vi "Sub Routing program.vi"(4 "Load Graph":refnum<vi>, 5 "Image":refnum<vi>, 6 "Test Name":refnum<vi>, 7 "FeedBack Channel":string[](array[string]), 8 "error in (no error)":errorcluster, 9 "Feature Step Enable":T1(array[cluster]), 10 "Table":refnum<vi>, 11 "queue Out in":refnum<queue>) -> (0 "error out":errorcluster, 1 "Error":bool, 2 "reference out":refnum<vi>, 3 "Queue out":refnum<queue>)   [LabVIEW 2015]
uses:
  Test  enqueue/AutoTest seq.ctl
  Galobal variable_TI.vi
panel:
  out "2D Picture 2":picture
  out "error out 2":errorcluster
  out "2D Picture":picture
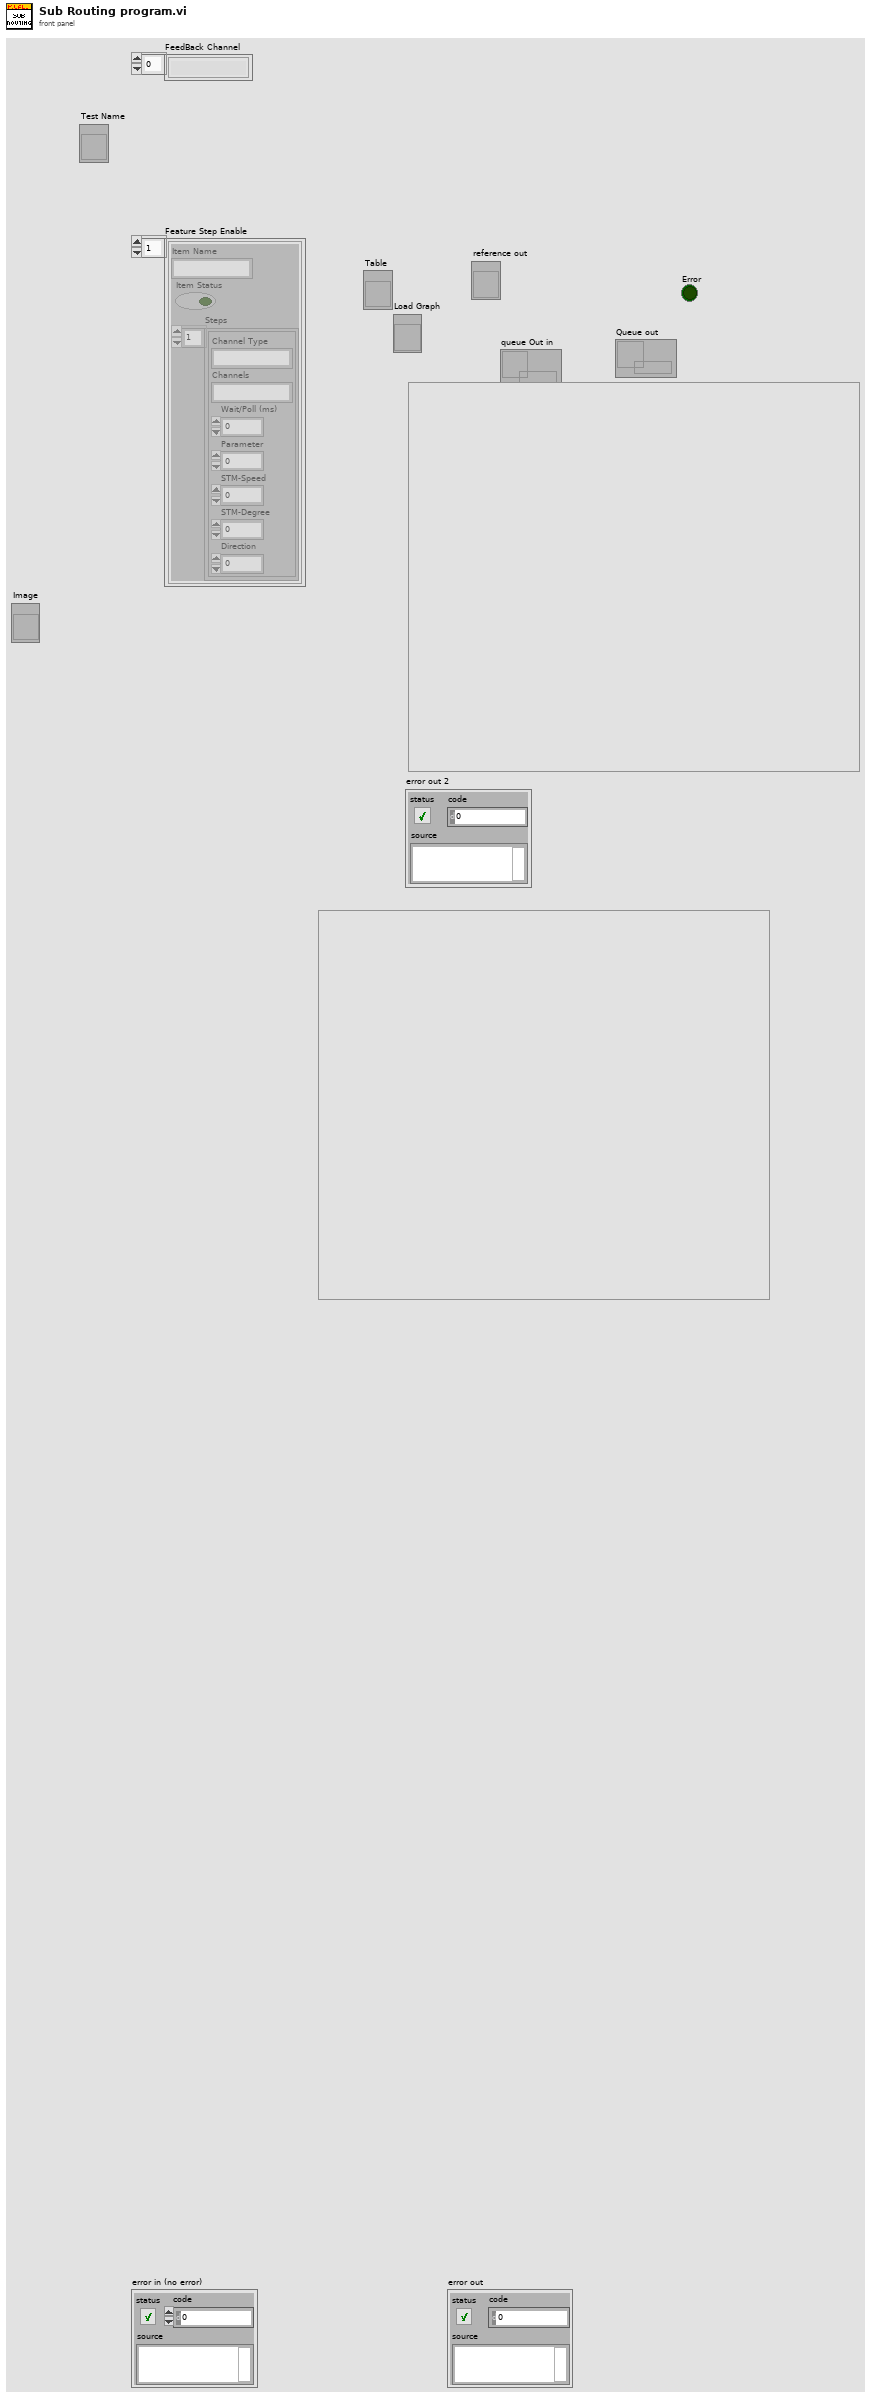
[diagram p1: front panel]
types:
  T1 = cluster{"Item Name":string, "Item Status":bool, "Steps":cluster{"Channel Type":string, "Channels":string, "Wait/Poll (ms)":u32, "Parameter":u8, "STM-Speed":i32, "STM-Degree":u32, "Direction":u8}[]}[]
  T2 = cluster{"Zoom Factor":sgl, "Horizontal position":sgl, "Vertical position":sgl}[]
  T3 = cluster{"Channel Type":string, "Channels":string, "Wait/Poll (ms)":u32, "Parameter":u8, "STM-Speed":i32, "STM-Degree":u32, "Direction":u8}[]
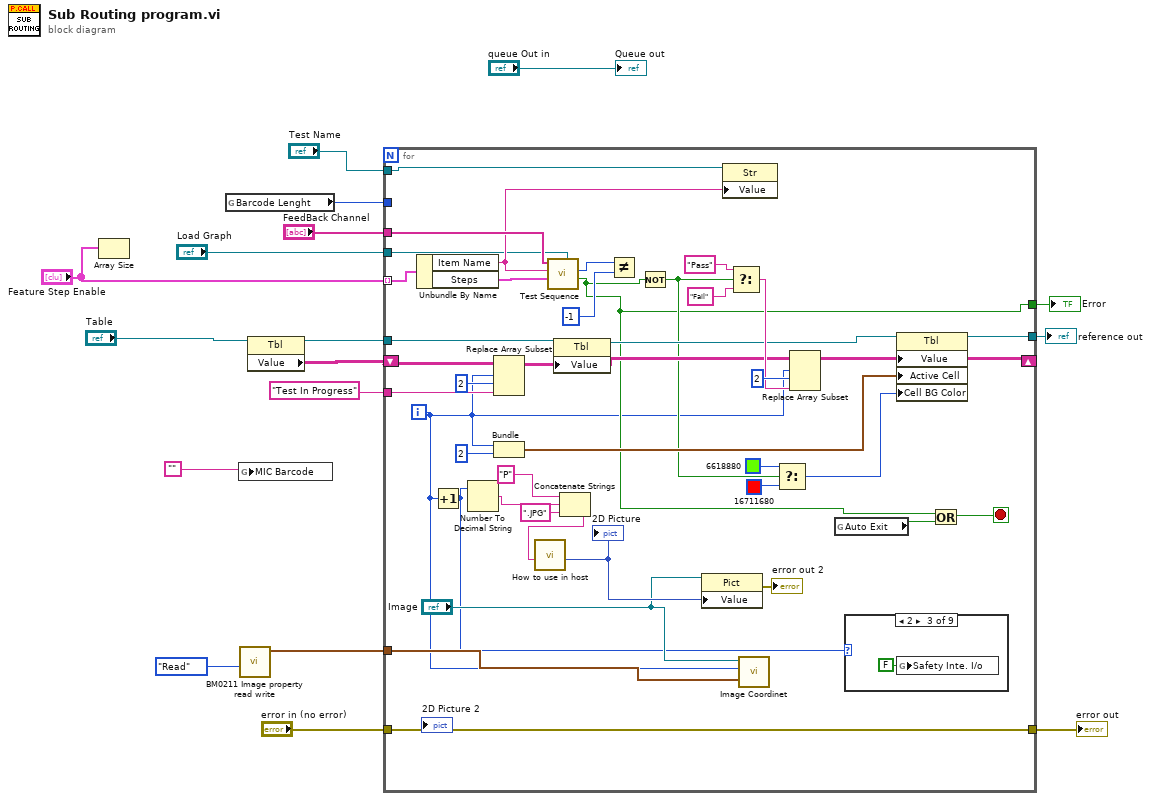
[diagram p0: block diagram]
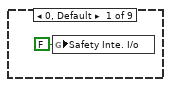
[diagram p2: hidden frame]
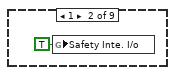
[diagram p3: hidden frame]
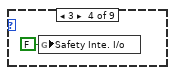
[diagram p4: hidden frame]
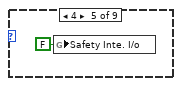
[diagram p5: hidden frame]
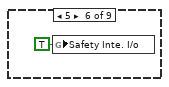
[diagram p6: hidden frame]
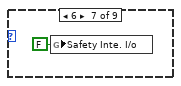
[diagram p7: hidden frame]
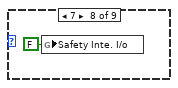
[diagram p8: hidden frame]
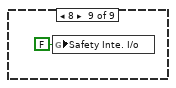
[diagram p9: hidden frame]
diagram:
  n1 = Array Size(array="Feature Step Enable") -> ()  [unwired: 1 out]
  n2 = global read "Galobal variable_TI.vi" "Barcode Lenght"() -> (w16:i32)
  n3 = global write "Galobal variable_TI.vi" "MIC Barcode"("") -> ()
  n4 = call "BM0211 Image property read write.vi"("Read write"=enum16{"write", "Read"}."Read") -> ("Out"=w3:T2)  [unwired: 9 in, 1 out]
  n5 = property class="Tbl"(reference="Table") -> (reference out=w10:refnum<vi>, "Value"=w13:string[][])  [unwired: 1 in, 1 out]
  n6 = for {
    tunnel: "Feature Step Enable" -> [w57] mode=indexing
    tunnel: "FeedBack Channel" -> [w54]
    tunnel: w16 -> [_]
    shift-right: [w38] -> _
    shift-left: w13 -> [w50]
    tunnel: "Test In Progress" ("new element/subarray") -> [w49]
    tunnel: w10 -> [w48]
    tunnel: [w39] -> w9
    tunnel: "error in (no error)" -> [w37]
    tunnel: [w37] -> w7
    tunnel: [w32] -> w6
    tunnel: "Test Name" -> [w31]
    tunnel: w3 -> [w23]
    tunnel: "Load Graph" -> [w20]
    i -> [w19]
    stop <- w21 stop-if-true
    n7 = Unbundle By Name(w57) -> ("Item Name"=w30:string, "Steps"=w53:T3)
    n8 = Increment(x=w19) -> (x+1=w18:i32)
    n9 = Number To Decimal String(number=w18) -> (decimal integer string=w26:string)  [unwired: 1 in]
    n10 = Replace Array Subset(array=w50, new element=w49, index (row)=w19, index (col)=2 ("disabled index (col)")) -> (w45:string[][])
    n11 = Bundle(w19, 2) -> (w44:cluster{i32, i32})  [unwired: 1 in]
    n12 = call "Test Sequence.vi"("FeedBack Channel"=w54, "Test Name"=w30, "Steps"=w53, "WFGraph Refnum"=w20) -> ("Out"=w36:i32, "Condition"=w32:bool)  [unwired: 3 in, 1 out]
    n13 = property class="Tbl"(reference=w48, "Value"=w45) -> (reference out=w40:refnum<vi>)  [unwired: 1 in, 1 out]
    n14 = Concatenate Strings("P" ("string"), w26, ".JPG" ("string")) -> (w25:string)
    n15 = call "How to use in host.vi"("element"=w25) -> ("2D Picture"=w29:picture)  [unwired: 9 in, 1 out]
    "2D Picture" <- w29
    n16 = Not Equal?(x=w36, y=-1) -> ()  [unwired: 1 out]
    n17 = Not(x=w32) -> (.not. x?=w33:bool)
    n18 = property class="Pict"(reference="Image", "Value"=w29) -> (error out=→"error out 2":errorcluster)  [unwired: 1 in, 1 out]
    n19 = property class="Str"(reference=w31, "Value"=w30) -> ()  [unwired: 1 in, 2 out]
    n20 = Select(t="Pass", s=w33, f="Fail") -> (s? t:f=w46:string)
    n21 = call "Image Coordinet.vi"("Out"=w23, "index of element"=w19, "Picture in"="Image") -> ()  [unwired: 9 in]
    n22 = Select(t=u32 6618880 ("Color Box"), s=w33, f=u32 16711680 ("Color Box")) -> (s? t:f=w41:u32)
    n23 = Replace Array Subset(array=w45, new element=w46, index (row)=w19, index (col)=2 ("disabled index (col)")) -> (w38:string[][])
    n24 = global read "Galobal variable_TI.vi" "Auto Exit"() -> (w34:bool)
    n25 = case shown="2" w18 {
      frame 0, Default {
        n26 = global write "Galobal variable_TI.vi" "Safety Inte. I/o"(FALSE ("Safety Inte. I/o")) -> ()
      }
      frame 1 {
        n27 = global write "Galobal variable_TI.vi" "Safety Inte. I/o"(TRUE ("Safety Inte. I/o")) -> ()
      }
      frame 2 {
        n28 = global write "Galobal variable_TI.vi" "Safety Inte. I/o"(FALSE ("Safety Inte. I/o")) -> ()
      }
      frame 3 {
        n29 = global write "Galobal variable_TI.vi" "Safety Inte. I/o"(FALSE ("Safety Inte. I/o")) -> ()
      }
      frame 4 {
        n30 = global write "Galobal variable_TI.vi" "Safety Inte. I/o"(FALSE ("Safety Inte. I/o")) -> ()
      }
      frame 5 {
        n31 = global write "Galobal variable_TI.vi" "Safety Inte. I/o"(TRUE ("Safety Inte. I/o")) -> ()
      }
      frame 6 {
        n32 = global write "Galobal variable_TI.vi" "Safety Inte. I/o"(FALSE ("Safety Inte. I/o")) -> ()
      }
      frame 7 {
        n33 = global write "Galobal variable_TI.vi" "Safety Inte. I/o"(FALSE ("Safety Inte. I/o")) -> ()
      }
      frame 8 {
        n34 = global write "Galobal variable_TI.vi" "Safety Inte. I/o"(FALSE ("Safety Inte. I/o")) -> ()
      }
    }
    n35 = property class="Tbl"(reference=w40, "Value"=w38, "Active Cell"=w44, "Cell BG Color"=w41) -> (reference out=w39:refnum<vi>)  [unwired: 1 in, 1 out]
    n36 = Or(x=w32, y=w34) -> (x .or. y?=w21:bool)
  }
  "error out" <- w7
  "reference out" <- w9
  "Error" <- w6
  "Queue out" <- "queue Out in"
